vi "Proxy_Init.vi"(8 "error in (no error)":errorcluster, 10 "Serial Options.Timeout (ms)":i32, 11 "VISA Refnum in":refnum<visa-resource-name>) -> (0 "error out":errorcluster, 3 "VISA Refnum out":refnum<visa-resource-name>)   [LabVIEW 2019]
uses:
  <vilib>/Instr/_visa.llb/VISA Configure Serial Port (Instr).vi
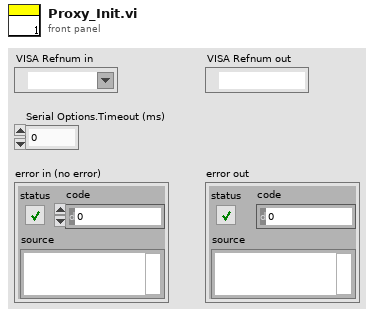
[diagram p1: front panel]
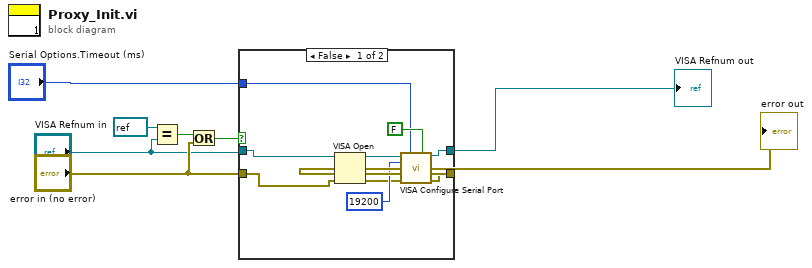
[diagram p0: block diagram]
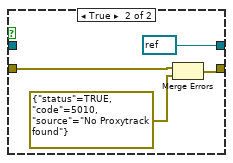
[diagram p2: hidden frame]
diagram:
  n1 = Equal?(x=refnum<visa-resource-name> refnum ("VISA resource out"), y="VISA Refnum in") -> (x = y?=w6:bool)
  n2 = Or(x=w6, y="error in (no error)") -> (x .or. y?=w8:bool)
  n3 = case shown="False" w8 {
    tunnel: "error in (no error)" -> [w13 w19]
    tunnel: "VISA Refnum in" -> [w9 _]
    tunnel: [w12 w18] -> w2
    tunnel: [w11 refnum<visa-resource-name> refnum ("VISA resource name out")] -> w1
    tunnel: "Serial Options.Timeout (ms)" -> [w10 _]
    frame False {
      n4 = VISA Open(error in (no error)=w13, VISA resource name=w9) -> (VISA resource name=w15:refnum<visa-resource-name>, error out=w14:errorcluster)  [unwired: 3 in]
      n5 = call-poly "VISA Configure Serial Port"("VISA resource name"=w15, "timeout (10sec)"=w10, "Enable Termination\nChar (T)"=FALSE ("Enable Termination\nChar (T)"), "baud rate (9600)"=u32 19200, "error in (no error)"=w14) -> ("VISA resource name out"=w11:refnum<visa-resource-name>, "error out"=w12:errorcluster)  [unwired: 9 in]
    }
    frame True {
      n6 = Merge Errors(w19, errorcluster {"status"=TRUE, "code"=5010, "source"="No Proxytrack found"} ("error out")) -> (w18:errorcluster)
    }
  }
  "error out" <- w2
  "VISA Refnum out" <- w1
